vi "Get Result Handler.vi"(8 "error in (no error)":errorcluster, 10 "Result":T1, 11 "Sequence in":refnum<class "Sequence.lvclass">) -> (0 "error out":errorcluster, 2 "Handler":refnum<class "Step.lvclass">, 3 "Sequence out":refnum<class "Sequence.lvclass">)   [LabVIEW 2020, in "Tester.lvlib" / "Sequence.lvclass"]
uses:
  Sequence.lvclass
  Results/Result.ctl
  Step/Step.lvclass
  Sequence.lvclass/Sequence.ctl
  <vilib>/Utility/error.llb/Error Cluster From Error Code.vi
  <vilib>/ErrorRing/Error Ring.xnode
  Results/Results.lvclass
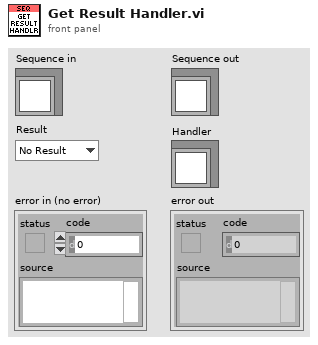
[diagram p1: front panel]
types:
  T1 = typedef "Tester.lvlib/Results.lvclass/Result.ctl" = enum16{"No Result", "Pass", "Fail", "Error", "Abort"}
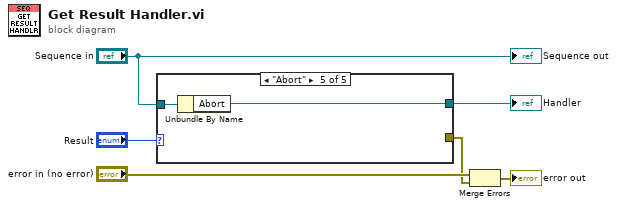
[diagram p0: block diagram]
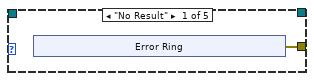
[diagram p2: hidden frame]
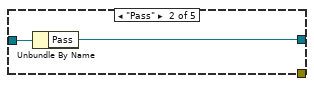
[diagram p3: hidden frame]
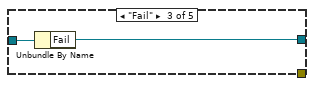
[diagram p4: hidden frame]
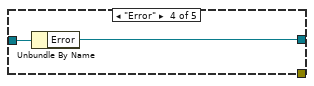
[diagram p5: hidden frame]
diagram:
  n1 = case shown="\"Abort\"" "Result" {
    tunnel: [w7 _ _ _ _] -> w3
    tunnel: "Sequence in" -> [_ w13 w15 w17 w19]
    tunnel: [_ w12 w14 w16 w18] -> w1
    frame "No Result" {
      n2 = xnode "Error Ring"() -> ("error out"=w7:errorcluster)
    }
    frame "Pass" {
      n3 = Unbundle By Name(w13) -> ("Pass"=w12:refnum<class "Step.lvclass">)
    }
    frame "Fail" {
      n4 = Unbundle By Name(w15) -> ("Fail"=w14:refnum<class "Step.lvclass">)
    }
    frame "Error" {
      n5 = Unbundle By Name(w17) -> ("Error"=w16:refnum<class "Step.lvclass">)
    }
    frame "Abort" {
      n6 = Unbundle By Name(w19) -> ("Abort"=w18:refnum<class "Step.lvclass">)
    }
  }
  "Handler" <- w1
  n7 = Merge Errors("error in (no error)", w3) -> (→"error out":errorcluster)
  "Sequence out" <- "Sequence in"
